vi "DDS_client_pulse_sequence.vi"() -> ()   [LabVIEW 2012]
uses:
  <userlib>/LabRAD/internal/Build Packet SubVIs/Build Packet by Name.vi
  <userlib>/LabRAD/internal/Simple Request SubVIs/Simple Request by Name.vi
panel:
  in  "Iterations":u32
  in  "DDS Pulses":T1(array[cluster])
  in  "update":bool
  out "client ID":u32
  out "welcome message":string
  in  "manager":T2={"address"="localhost", "port"=7682, "password"=""}
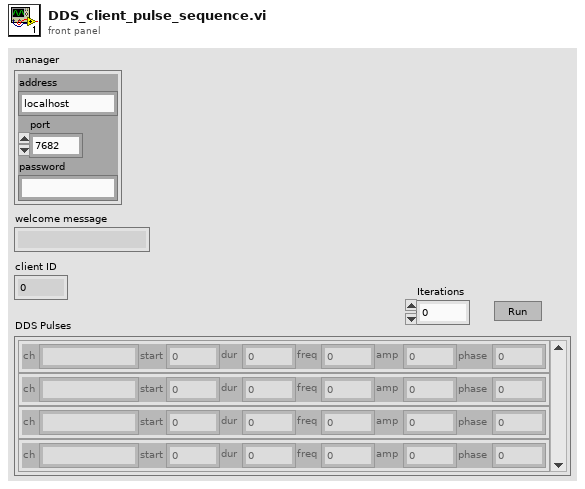
[diagram p1: front panel]
types:
  T1 = cluster{"ch":string, "start":dbl, "dur":dbl, "freq":dbl, "amp":dbl, "phase":dbl}[]
  T2 = cluster{"address":string, "port":u16, "password":string}
  T3 = cluster{"Setting":cluster{"ID":u32, "Name":string}, "Type Tag":string, "Data":string}[]
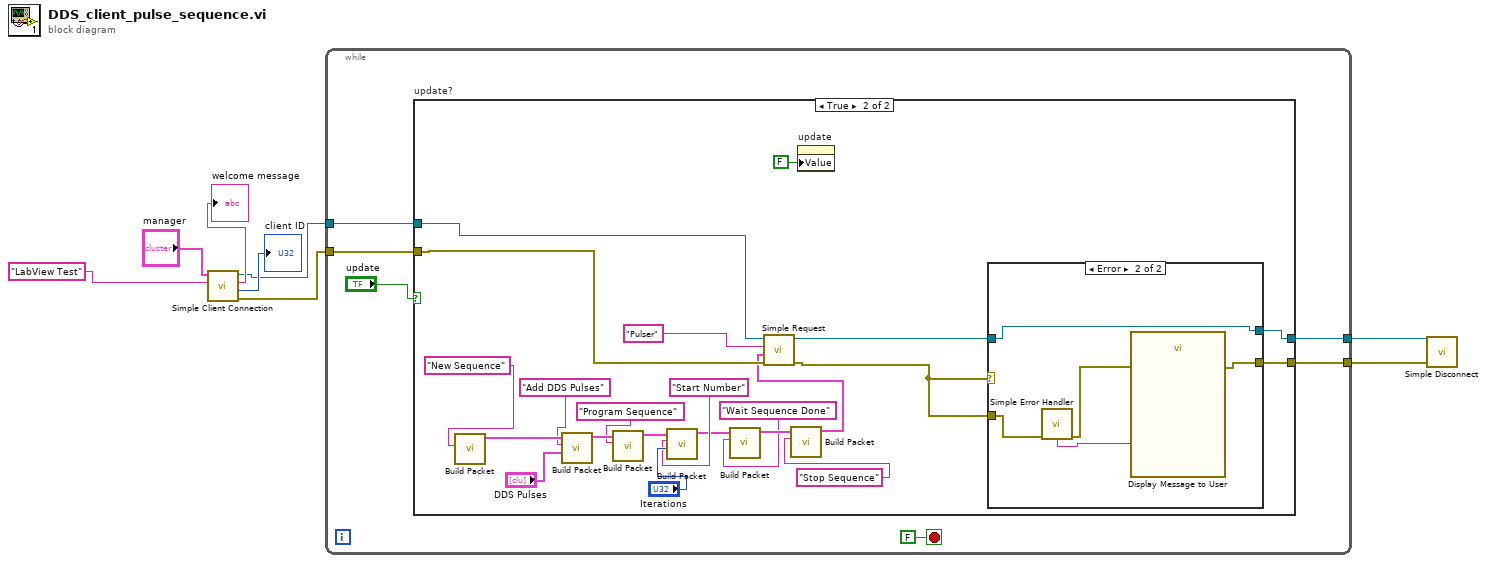
[diagram p0: block diagram]
diagram:
  n1 = call <userlib>:"Simple Client Connection.vi"("connection name (LabVIEW Client)"="LabView Test", "manager"="manager") -> ("error out"=w4:errorcluster, "client ID"=→"client ID":u32, "welcome message"=→"welcome message":string, "connection ID out"=w3:refnum<k5>)  [unwired: 2 in]
  n2 = while {
    tunnel: w4 -> [w12]
    tunnel: w3 -> [w11]
    tunnel: [w10] -> w2
    tunnel: [w9] -> w1
    stop <- FALSE stop-if-true
    n3 = case "update?" shown="True" "update" {
      tunnel: w12 -> [w15 w35]
      tunnel: w11 -> [w16 w36]
      tunnel: [w16 w24] -> w10
      tunnel: [w15 w25] -> w9
      frame False {
      }
      frame True {
        n4 = call-poly <userlib>:"Build Packet.vi"("setting"="New Sequence") -> ("appended records"=w32:T3)  [unwired: 7 in, 2 out]
        n5 = call-poly <userlib>:"Build Packet.vi"("data (empty)"="DDS Pulses", "setting"="Add DDS Pulses", "records (empty)"=w32) -> ("appended records"=w30:T3)  [unwired: 5 in, 2 out]
        n6 = call-poly <userlib>:"Build Packet.vi"("setting"="Program Sequence", "records (empty)"=w30) -> ("appended records"=w28:T3)  [unwired: 6 in, 2 out]
        n7 = call-poly <userlib>:"Build Packet.vi"("data (empty)"="Iterations", "setting"="Start Number", "records (empty)"=w28) -> ("appended records"=w21:T3)  [unwired: 5 in, 2 out]
        n8 = call-poly <userlib>:"Build Packet.vi"("setting"="Wait Sequence Done", "records (empty)"=w21) -> ("appended records"=w20:T3)  [unwired: 6 in, 2 out]
        n9 = call-poly <userlib>:"Build Packet.vi"("setting"="Stop Sequence", "records (empty)"=w20) -> ("appended records"=w17:T3)  [unwired: 6 in, 2 out]
        n10 = call-poly <userlib>:"Simple Request.vi"("error in (no error)"=w35, "records in (empty)"=w17, "target (Manager)"="Pulser", "connection ID"=w36) -> ("error out"=w26:errorcluster, "connection ID out"=w23:refnum<k5>)  [unwired: 2 in, 2 out]
        n11 = property on="update" class="Bool (strict)"("Value"=FALSE ("update")) -> ()  [unwired: 2 in, 2 out]
        n12 = case shown="Error" w26 {
          tunnel: w26 -> [w40 w45]
          tunnel: [w40 w42] -> w25
          tunnel: [w39 w41] -> w24
          tunnel: w23 -> [w39 w41]
          frame No Error {
          }
          frame Error {
            n13 = call <vilib>:"Simple Error Handler.vi"("error in (no error)"=w45) -> ("error out"=w43:errorcluster, "message"=w44:string)  [unwired: 4 in, 3 out]
            n14 = call "Display Message to User"("error in (no error)"=w43, "Message"=w44) -> ("error out"=w42:errorcluster)  [unwired: 8 in, 1 out]
          }
        }
      }
    }
  }
  n15 = call <userlib>:"Simple Disconnect.vi"("error in (no error)"=w1, "connection ID"=w2) -> ()  [unwired: 5 in, 1 out]
